vi "MQTT_ConnAck_Send.vi"(8 "error in (no error)":errorcluster, 10 "Conn Return Code":T2=enum."Connection refused: not authorized", 11 "SSL_Connection":T1) -> (0 "error out":errorcluster, 2 "ConnAck Message":u8[](array[numeric]) format="%x", 3 "SSL_Connection":T1)   [LabVIEW 2018, in "AWS_IoT.lvlib"]
uses:
  AWS_IoT.lvlib
  Controls/Connection_Return_Codes.ctl
  Controls/SSL_Connection.ctl
  Controls/MessageType.ctl
  Controls/Retain_Flag.ctl
  Controls/DUP_Flag.ctl
  Controls/QoS.ctl
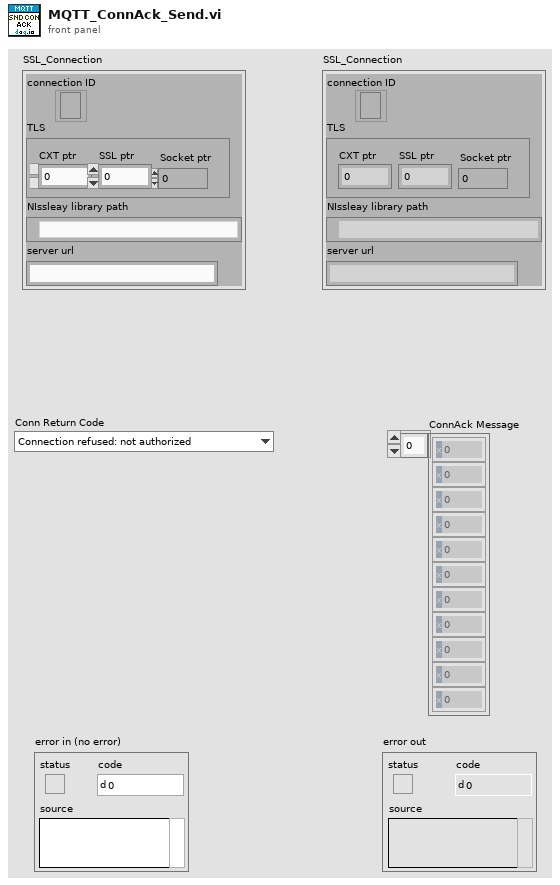
[diagram p1: front panel]
types:
  T1 = typedef "AWS_IoT.lvlib/SSL_Connection.ctl" = cluster{"connection ID":refnum<k5>, "TLS":cluster{"CXT ptr":i32, "SSL ptr":i32, "Socket ptr":i32}, "NIssleay library path":path, "server url":string}
  T2 = typedef "AWS_IoT.lvlib/Connection_Return_Codes.ctl" = enum16{"Connection accepted", "Connection refused: unacceptable protocol version", "Connection refused: identifier rejected", "Connection refused: Server unavailable", "Connection refused: bad user name or password", "Connection refused: not authorized"}
  T3 = typedef "AWS_IoT.lvlib/QoS.ctl" = enum8{"At most once", "At least once", "Exactly once", "Reserved"}
  T4 = typedef "AWS_IoT.lvlib/DUP_Flag.ctl" = bool
  T5 = typedef "AWS_IoT.lvlib/Retain_Flag.ctl" = bool
  T6 = typedef "AWS_IoT.lvlib/MessageType.ctl" = enum32{"Reserved", "CONNECT", "CONNACK", "PUBLISH", "PUBACK", "PUBREC", "PUBREL", "PUBCOMP", "SUBSCRIBE", "SUBACK", "UNSUBSCRIBE", "UNSUBACK", "PINGREQ", "PINGRESP", "DISCONNECT", "Reserved2"}
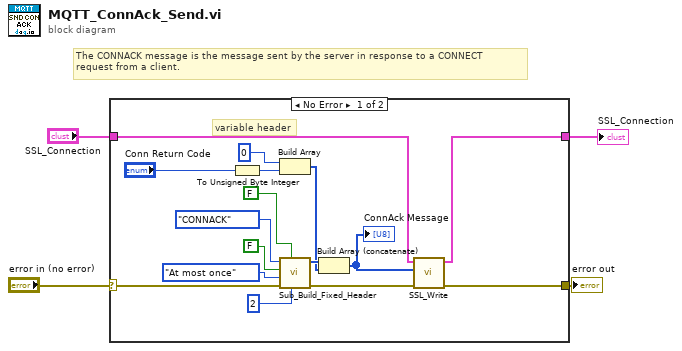
[diagram p0: block diagram]
diagram:
  # "The CONNACK message is the message sent by the server in response to a CONNECT\nrequest from a client."
  n1 = case shown="No Error" "error in (no error)" {
    selector: "error in (no error)" -> [w14 w22]
    tunnel: [w7 w22] -> w3
    tunnel: "SSL_Connection" -> [w6 w21]
    tunnel: [w5 w21] -> w1
    frame No Error {
      # "variable header"
      n2 = To Unsigned Byte Integer(number="Conn Return Code") -> (unsigned 8bit integer=w11:u8)
      n3 = Build Array(u8 0 ("element"), w11) -> (w13:u8[])
      n4 = call "Sub_Build_Fixed_Header.vi"("Remaining Length"=u32 2, "Retain"=T5 FALSE, "error in (no error)"=w14, "QoS"=QoS."At most once", "DUP"=T4 FALSE, "MessageType"=MessageType."CONNACK") -> ("error out"=w8:errorcluster, "Fixed Header"=w19:u8[])  [unwired: 4 in]
      n5 = Build Array (concatenate)(w19, w13) -> (w9:u8[])
      "ConnAck Message" <- w9
      n6 = call "SSL_Write.vi"("error in (no error)"=w8, "data in"=w9, "SSL_Connection"=w6) -> ("error out"=w7:errorcluster, "SSL_Connection"=w5:T1)  [unwired: 7 in]
    }
    frame Error {
    }
  }
  "error out" <- w3
  "SSL_Connection" <- w1
